vi "cm_Channel Monitor Event Detect.vi"(8 "error in (no error)":errorcluster, 10 "New Value":T1[](array[typedef]) {"Current Level" scale=0.0..1.0; "Peak Level" scale=0.0..1.0}, 11 "Old Value":T1[](array[typedef]) {"Current Level" scale=0.0..1.0; "Peak Level" scale=0.0..1.0}) -> (0 "error out":errorcluster, 1 "Channel":i32, 2 "Button":string, 3 "Updated Value":T1[](array[typedef]) {"Current Level" scale=0.0..1.0; "Peak Level" scale=0.0..1.0})   [LabVIEW 2012, in "Channel Monitor.xctl"]
uses:
  Channel Monitor.xctl
  TypeDef/cm_Channel Indicator.ctl
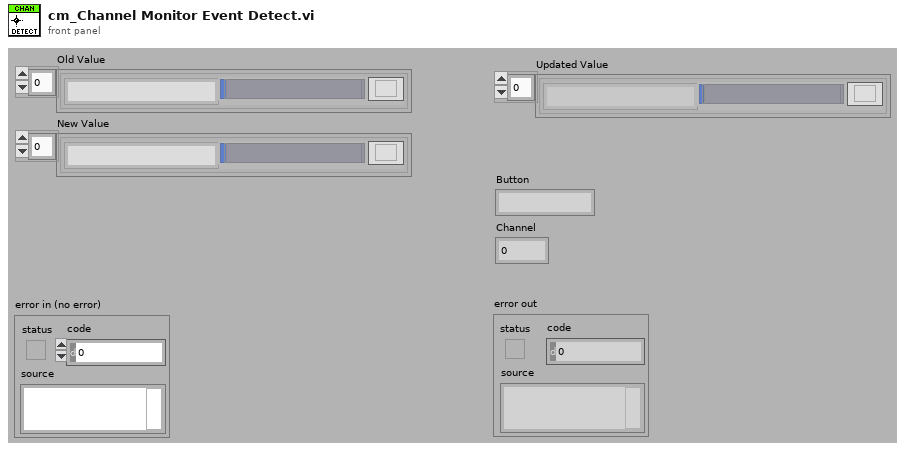
[diagram p1: front panel]
types:
  T1 = typedef "Channel Monitor.xctl/cm_Channel Indicator.ctl" = cluster{"Channel Name":string, "TimeDomain":bool, "Peak Level":dbl, "Current Level":dbl}
  T2 = cluster{"Channel Name":bool, "Level":bool, "TimeDomain":bool, "TimeDomain 2":bool}
  T3 = cluster{"Channel Name":bool, "TimeDomain":bool, "Peak Level":bool, "Current Level":bool}[]
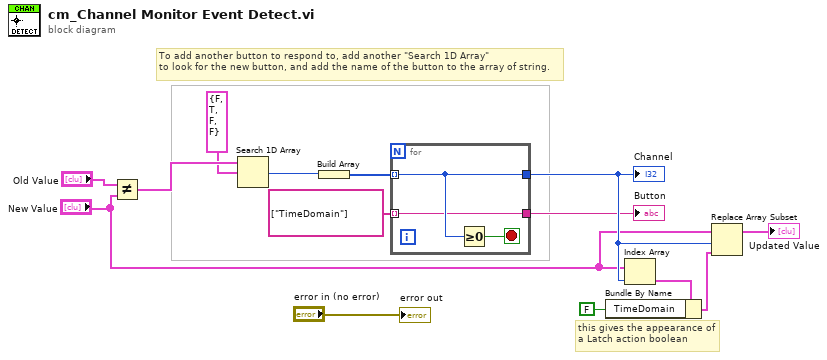
[diagram p0: block diagram]
diagram:
  # "this gives the appearance of a Latch action boolean"
  # "To add another button to respond to, add another \"Search 1D Array\"\nto look for the new button, and add the name of the button to the array of string."
  n1 = Not Equal?(x="Old Value", y="New Value") -> (x != y?=w6:T3)
  n2 = Search 1D Array(1D array=w6, element=T2 {"Channel Name"=FALSE, "Level"=TRUE, "TimeDomain"=FALSE, "TimeDomain 2"=FALSE}) -> (index of element=w7:i32)  [unwired: 1 in]
  n3 = Build Array(w7) -> (w8:i32[])
  n4 = for {
    tunnel: w8 -> [w16] mode=indexing
    tunnel: [w16] -> w13
    tunnel: string[] ["TimeDomain"] -> [w15] mode=indexing
    tunnel: [w15] -> w10
    stop <- w17 stop-if-true
    n5 = Greater Or Equal To 0?(x=w16) -> (x >= 0?=w17:bool)
  }
  "Channel" <- w13
  "Button" <- w10
  n6 = Index Array(array="New Value", index=w13) -> (element=w11:T1)
  n7 = Bundle By Name(cluster=w11, "TimeDomain"=FALSE) -> (w14:T1)
  n8 = Replace Array Subset(array="New Value", new element=w14, index=w13) -> (→"Updated Value":T1[])
  "error out" <- "error in (no error)"
